vi "Crear_Variant.vi"() -> ()   [LabVIEW 2016]
panel:
  out "duplicate variant":variant
  in  "String":string
  in  "Boolean":bool
  in  "Numeric Control":dbl
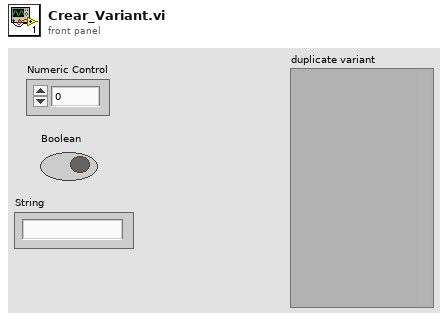
[diagram p1: front panel]
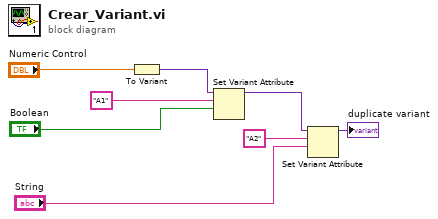
[diagram p0: block diagram]
diagram:
  n1 = To Variant(anything="Numeric Control") -> (Variant=w8:variant)
  n2 = Set Variant Attribute(Variant=w8, name="A1", value="Boolean") -> (Variant out=w4:variant)  [unwired: 1 in, 2 out]
  n3 = Set Variant Attribute(Variant=w4, name="A2", value="String") -> (Variant out=→"duplicate variant":variant)  [unwired: 1 in, 2 out]
